vi "ReadKeyboardCommand.vi"(3 "handle":i32, 5 "Motion #":u32, 6 "Enable\n(True)":bool) -> (0 "Enable Move\n(TRUE)":bool, 1 "Move size (mm)":dbl, 2 "Axis":enum16{"X", "Y"}(ring))   [LabVIEW 2011]
uses:
  MCL libraries/MicroDrive.dll
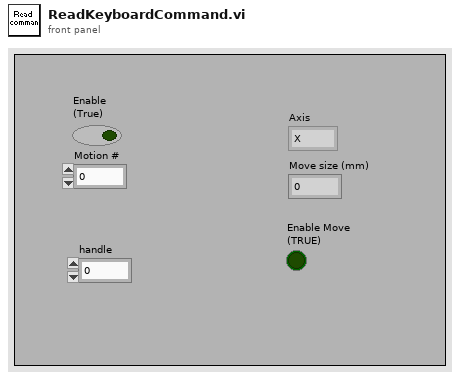
[diagram p1: front panel]
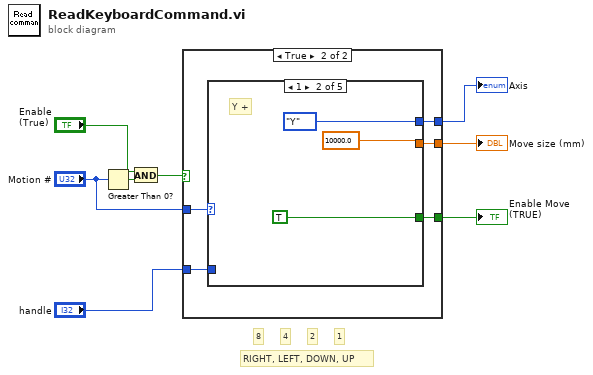
[diagram p0: block diagram]
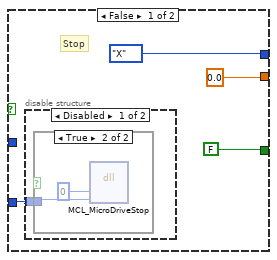
[diagram p2: hidden frame]
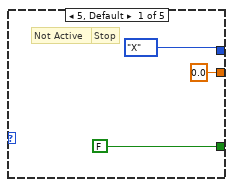
[diagram p5: hidden frame]
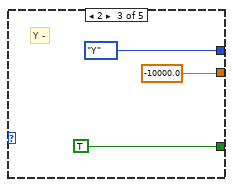
[diagram p6: hidden frame]
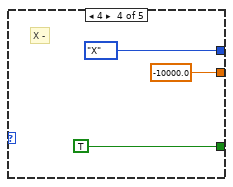
[diagram p7: hidden frame]
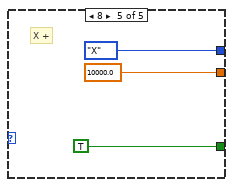
[diagram p8: hidden frame]
diagram:
  # "8"
  # "4"
  # "2"
  # "1"
  # "RIGHT, LEFT, DOWN, UP"
  n1 = Greater Than 0?(x="Motion #") -> (x > 0?=w8:bool)
  n2 = And(x="Enable\n(True)", y=w8) -> (x .and. y?=w7:bool)
  n3 = case shown="True" w7 {
    tunnel: [FALSE w20] -> w1
    tunnel: [enum16{"X", "Y"}."X" ("Axis 2") w19] -> w3
    tunnel: "handle" -> [w10 w18]
    tunnel: "Motion #" -> [_ w17]
    tunnel: [0.0 ("Move size (mm)") w16] -> w2
    frame False {
      # "Stop"
      n4 = disable-structure shown="Disabled" {
        disable-tunnel: w10 -> [w13 _]
        frame Disabled {
          n5 = case shown="True" {
            selector: _ -> [_ _]
            tunnel: w13 -> [_ w14]
            frame False {
            }
            frame True {
              n6 = dll-call lib="C:/Labview code/2D photogate/MCL libraries/MicroDrive.dll" fn="MCL_MicroDriveStop"("status"=0, "handle"=w14) -> ()  [unwired: 4 in, 4 out]
            }
          }
        }
        frame Enabled {
        }
      }
    }
    frame True {
      n7 = case shown="1" w17 {
        tunnel: w18 -> [_ _ _ _ _]
        tunnel: [FALSE TRUE TRUE TRUE TRUE] -> w20
        tunnel: [enum16{"X", "Y"}."X" ("Axis 2") enum16{"X", "Y"}."Y" ("Axis 2") enum16{"X", "Y"}."Y" ("Axis 2") enum16{"X", "Y"}."X" ("Axis 2") enum16{"X", "Y"}."X" ("Axis 2")] -> w19
        tunnel: [0.0 ("Move size (mm)") 10000.0 ("Move size (mm)") -10000.0 ("Move size (mm)") -10000.0 ("Move size (mm)") 10000.0 ("Move size (mm)")] -> w16
        frame 5, Default {
          # "Stop"
          # "Not Active"
        }
        frame 1 {
          # "Y +"
        }
        frame 2 {
          # "Y -"
        }
        frame 4 {
          # "X -"
        }
        frame 8 {
          # "X +"
        }
      }
    }
  }
  "Axis" <- w3
  "Move size (mm)" <- w2
  "Enable Move\n(TRUE)" <- w1
